vi "题目3.vi"(0 "温度单位":bool, 1 "停止":bool) -> (2 "温度计":dbl(slide) scale=0.0..260.0, 3 "字符串":string)   [LabVIEW 2017]
panel:
  # "°F"
  # "°C"
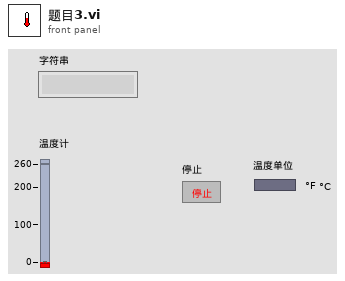
[diagram p1: front panel]
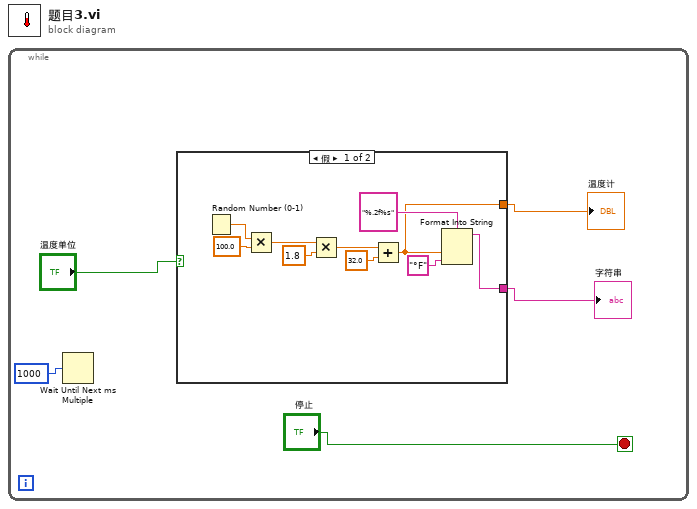
[diagram p0: block diagram]
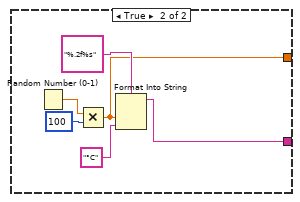
[diagram p2: hidden frame]
diagram:
  n1 = while {
    stop <- "停止" stop-if-true
    n2 = Wait Until Next ms Multiple(millisecond multiple=u32 1000 ("毫秒计时值")) -> ()  [unwired: 1 out]
    n3 = case shown="假" "温度单位" {
      tunnel: [w7 w17] -> w1
      tunnel: [w6 w16] -> w2
      frame False {
        n4 = Random Number (0-1)() -> (number: 0 to 1=w15:dbl)
        n5 = Multiply(x=w15, y=100.0) -> (x*y=w13:dbl)
        n6 = Multiply(x=w13, y=1.8) -> (x*y=w11:dbl)
        n7 = Add(x=w11, y=32.0) -> (x+y=w6:dbl)
        n8 = Format Into String(format string="%.2f%s", w6, "°F") -> (resulting string=w7:string)  [unwired: 2 in, 1 out]
      }
      frame True {
        n9 = Random Number (0-1)() -> (number: 0 to 1=w21:dbl)
        n10 = Multiply(x=w21, y=100) -> (x*y=w16:dbl)
        n11 = Format Into String ("格式化写入字符串")(format string="%.2f%s", w16, "°C") -> (resulting string=w17:string)  [unwired: 2 in, 1 out]
      }
    }
    "温度计" <- w2
    "字符串" <- w1
  }
